vi "PlayWithBitmap.vi"() -> ()   [LabVIEW 2014]
panel:
  out "80 by 80 array":u8[][](array[numeric])
  out "Every 6th red pixel value":u8[](array[numeric])
  out "Blue pixel values":u8[](array[numeric])
  out "Geen pixel values":u8[](array[numeric])
  out "Red pixel values":u8[](array[numeric])
  out "Red array size":dbl
  out "Image RGB values":u8[](array[numeric])
  # "Play with bitmap"
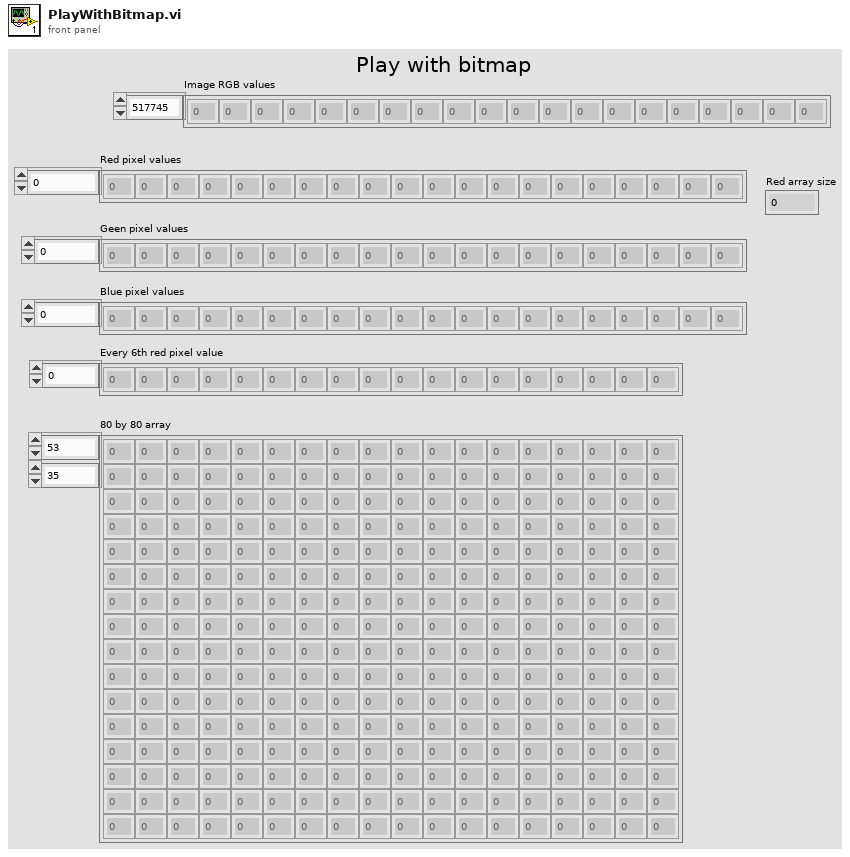
[diagram p1: front panel]
types:
  T1 = typedef "imagedata.ctl" = cluster{"image type":i32, "image depth":i32, "image":u8[], "mask":u8[], "colors":u32[], "Rectangle":cluster{"left":i16, "top":i16, "right":i16, "bottom":i16}}
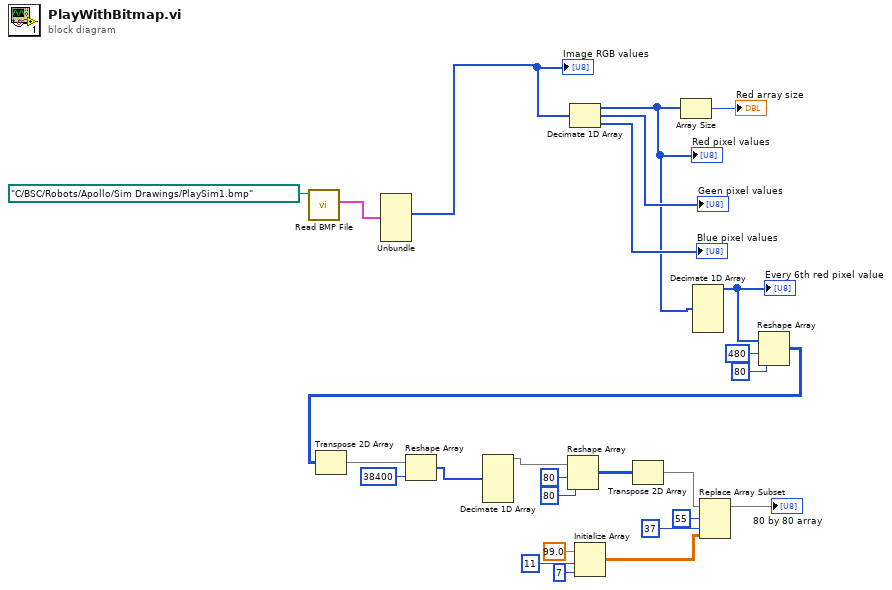
[diagram p0: block diagram]
diagram:
  n1 = call <vilib>:"Read BMP File.vi"("path to BMP file"=path "C:/BSC/Robots/Apollo/Sim Drawings/PlaySim1.bmp") -> ("image data"=w25:T1)  [unwired: 8 in, 2 out]
  n2 = Unbundle(w25) -> ("image"=w23:u8[])  [unwired: 5 out]
  "Image RGB values" <- w23
  n3 = Decimate 1D Array(w23) -> (w20:u8[], →"Geen pixel values":u8[], →"Blue pixel values":u8[])
  "Red pixel values" <- w20
  n4 = Initialize Array(99.0 ("element"), 11 ("dimension size"), 7 ("dimension size")) -> (w2:dbl[][])
  n5 = Array Size(array=w20) -> (size(s)=→"Red array size":i32)
  n6 = Decimate 1D Array(w20) -> (w19:u8[])  [unwired: 5 out]
  "Every 6th red pixel value" <- w19
  n7 = Reshape Array(w19, 480 ("dimension size"), 80 ("dimension size")) -> (w16:u8[][])
  n8 = Transpose 2D Array(2D array=w16) -> (transposed array=w15:u8[][])
  n9 = Reshape Array(w15, 38400 ("dimension size")) -> (w13:u8[])
  n10 = Decimate 1D Array(w13) -> (w12:u8[])  [unwired: 5 out]
  n11 = Reshape Array(w12, 80 ("dimension size"), 80 ("dimension size")) -> (w9:u8[][])
  n12 = Transpose 2D Array(2D array=w9) -> (transposed array=w8:u8[][])
  n13 = Replace Array Subset(array=w8, new element=w2, index (row)=55, index (col)=37 ("disabled index (col)")) -> (→"80 by 80 array":u8[][])
